vi "Close.vi"(8 "error in (no error)":errorcluster, 11 "PS Driver Actor in":refnum<class "PS Driver.lvclass">) -> (0 "error out":errorcluster, 3 "PS Driver Actor out":refnum<class "PS Driver.lvclass">)   [LabVIEW 2022 SP3, in "PS Driver.lvlib" / "PS Driver.lvclass"]
uses:
  PS Driver.lvclass
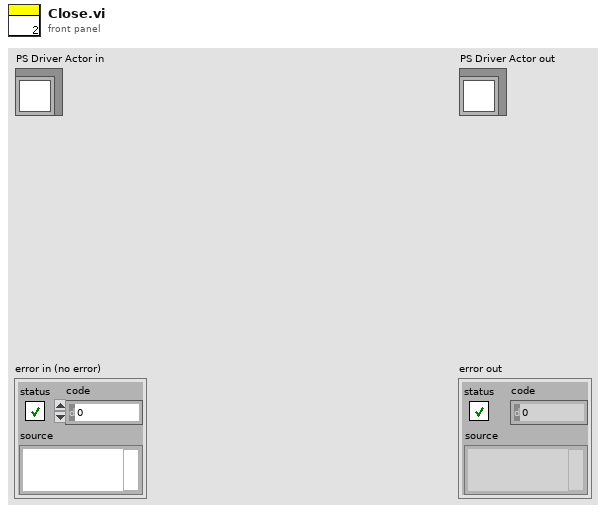
[diagram p1: front panel]
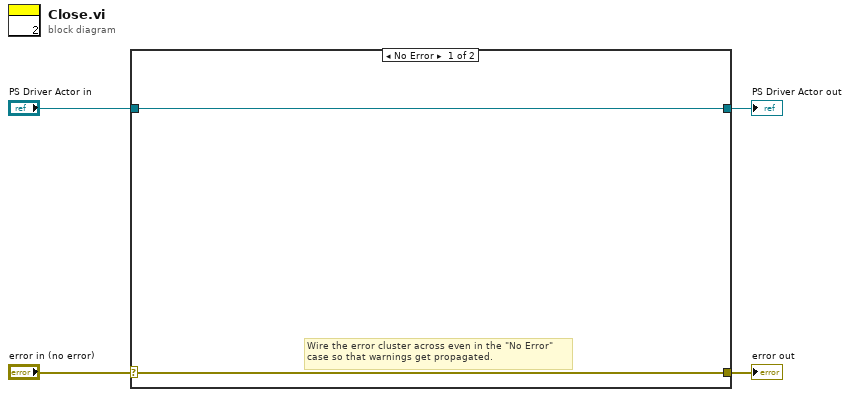
[diagram p0: block diagram]
diagram:
  n1 = case shown="No Error" "error in (no error)" {
    selector: "error in (no error)" -> [w5 w8]
    tunnel: [w5 w8] -> w3
    tunnel: [w6 w7] -> w1
    tunnel: "PS Driver Actor in" -> [w6 w7]
    frame No Error {
      # "Wire the error cluster across even in the \"No Error\"\ncase so that warnings get propagated."
    }
    frame Error {
    }
  }
  "error out" <- w3
  "PS Driver Actor out" <- w1
